vi "brookfield read external mode.vi"() -> ()   [LabVIEW 2019]
uses:
  <vilib>/Instr/_visa.llb/VISA Configure Serial Port (Instr).vi
panel:
  out "Conrtro Circuitry Enabled":bool
  out "Motor On":bool
  out "Motor Stopped":bool
  out "Auto-zero Complete":bool
  out "Motor Circuit Error":bool
  out "Diagnostics Error":bool
  out "Invalid Command Received":bool
  out "resulting string":string
  out "temp":dbl
  out "torque%":dbl
  out "length":i32
  out "read buffer":string
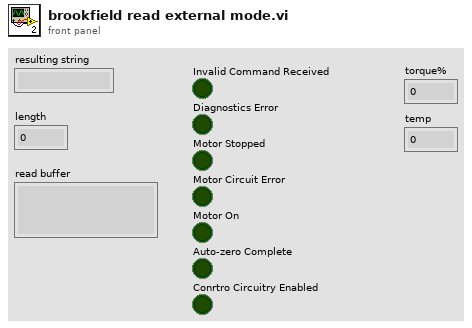
[diagram p1: front panel]
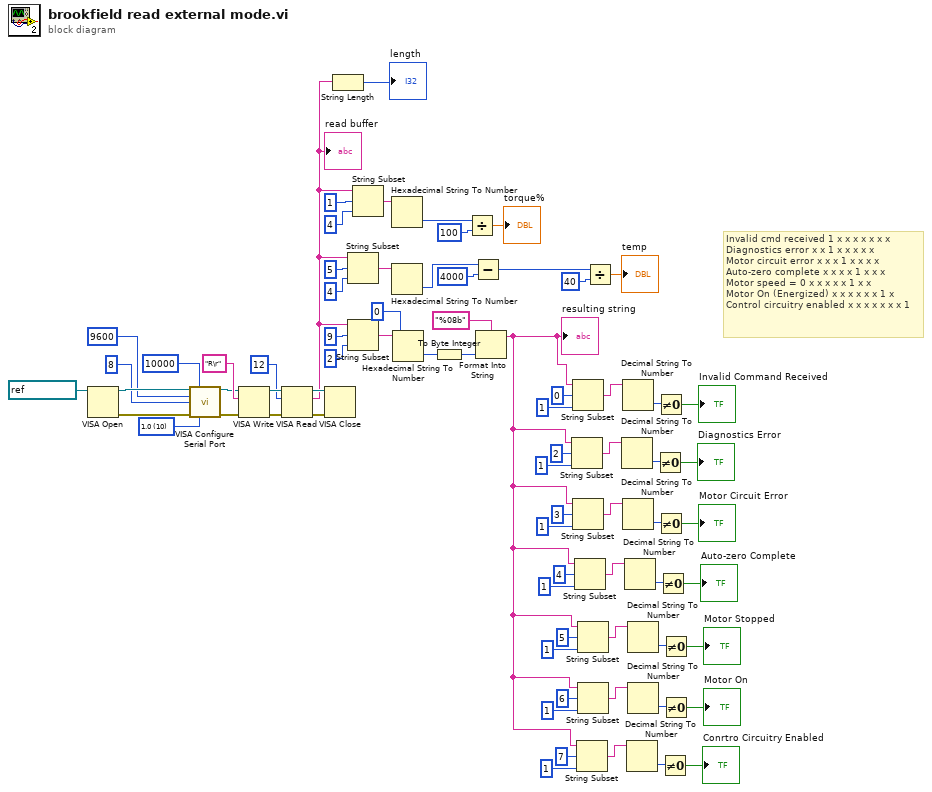
[diagram p0: block diagram]
diagram:
  w63 = u16 10 items=["1.0"=10, "1.5"=15, "2.0"=20] ("stop bits (10: 1 bit)")
  # "Invalid cmd received 1 x x x x x x x\nDiagnostics error x x 1 x x x x x\nMotor circuit error x x x 1 x x x x\nAuto-zero complete x x x x 1 x x x\nMotor speed = 0 x x x x x 1 x x\nMotor On (Energized) x x x x x x 1 x\nControl circuitry enabled x x x x x x x 1"
  n1 = VISA Open(VISA resource name=refnum<visa-resource-name> "COM11" ("Conductivity Port")) -> (VISA resource name=w67:refnum<visa-resource-name>, error out=w69:errorcluster)  [unwired: 4 in]
  n2 = call-poly "VISA Configure Serial Port"("VISA resource name"=w67, "timeout (10sec)"=u32 10000, "baud rate (9600)"=u32 9600, "data bits (8)"=u16 8, "error in (no error)"=w69, "stop bits (10: 1 bit)"=w63) -> ("VISA resource name out"=w62:refnum<visa-resource-name>, "error out"=w61:errorcluster)  [unwired: 8 in]
  n3 = VISA Write(VISA resource name=w62, write buffer="R\r", error in (no error)=w61) -> (VISA resource name out=w73:refnum<visa-resource-name>, error out=w72:errorcluster)  [unwired: 1 out]
  n4 = VISA Read(VISA resource name=w73, byte count=u32 12, error in (no error)=w72) -> (VISA resource name out=w60:refnum<visa-resource-name>, read buffer=w42:string, error out=w59:errorcluster)  [unwired: 1 out]
  "read buffer" <- w42
  n5 = VISA Close(VISA resource name=w60, error in (no error)=w59) -> ()  [unwired: 1 out]
  n6 = String Length(string=w42) -> (length=→"length":i32)
  n7 = String Subset(string=w42, offset (0)=5, length (rest)=4 ("length (rest)")) -> (substring=w49:string)
  n8 = String Subset(string=w42, offset (0)=9, length (rest)=2 ("length (rest)")) -> (substring=w41:string)
  n9 = String Subset(string=w42, offset (0)=1, length (rest)=4 ("length (rest)")) -> (substring=w56:string)
  n10 = Hexadecimal String To Number(string=w56) -> (number=w55:u32)  [unwired: 2 in, 1 out]
  n11 = Hexadecimal String To Number(string=w49) -> (number=w48:u32)  [unwired: 2 in, 1 out]
  n12 = Hexadecimal String To Number(string=w41, default (0uL)=u32 0 ("default (0 U32)")) -> (number=w32:u32)  [unwired: 1 in, 1 out]
  n13 = To Byte Integer(number=w32) -> (8bit integer=w33:i8)
  n14 = Divide(x=w55, y=u32 100) -> (x/y=→"torque%":dbl)
  n15 = Subtract(x=w48, y=u32 4000) -> (x-y=w46:u32)
  n16 = Format Into String(format string="%08b", w33) -> (resulting string=w1:string)  [unwired: 2 in, 1 out]
  "resulting string" <- w1
  n17 = String Subset(string=w1, offset (0)=2, length (rest)=1 ("length (rest)")) -> (substring=w29:string)
  n18 = String Subset(string=w1, offset (0)=0, length (rest)=1 ("length (rest)")) -> (substring=w37:string)
  n19 = String Subset(string=w1, offset (0)=3, length (rest)=1 ("length (rest)")) -> (substring=w24:string)
  n20 = String Subset(string=w1, offset (0)=4, length (rest)=1 ("length (rest)")) -> (substring=w19:string)
  n21 = String Subset(string=w1, offset (0)=7, length (rest)=1 ("length (rest)")) -> (substring=w4:string)
  n22 = String Subset(string=w1, offset (0)=5, length (rest)=1 ("length (rest)")) -> (substring=w14:string)
  n23 = String Subset(string=w1, offset (0)=6, length (rest)=1 ("length (rest)")) -> (substring=w9:string)
  n24 = Divide(x=w46, y=u32 40) -> (x/y=→"temp":dbl)
  n25 = Decimal String To Number(string=w29) -> (number=w30:i32)  [unwired: 2 in, 1 out]
  n26 = Decimal String To Number(string=w37) -> (number=w36:i32)  [unwired: 2 in, 1 out]
  n27 = Decimal String To Number(string=w24) -> (number=w23:i32)  [unwired: 2 in, 1 out]
  n28 = Decimal String To Number(string=w19) -> (number=w20:i32)  [unwired: 2 in, 1 out]
  n29 = Decimal String To Number(string=w4) -> (number=w3:i32)  [unwired: 2 in, 1 out]
  n30 = Decimal String To Number(string=w14) -> (number=w13:i32)  [unwired: 2 in, 1 out]
  n31 = Decimal String To Number(string=w9) -> (number=w10:i32)  [unwired: 2 in, 1 out]
  n32 = Not Equal To 0?(x=w30) -> (x != 0?=→"Diagnostics Error":bool)
  n33 = Not Equal To 0?(x=w36) -> (x != 0?=→"Invalid Command Received":bool)
  n34 = Not Equal To 0?(x=w23) -> (x != 0?=→"Motor Circuit Error":bool)
  n35 = Not Equal To 0?(x=w20) -> (x != 0?=→"Auto-zero Complete":bool)
  n36 = Not Equal To 0?(x=w3) -> (x != 0?=→"Conrtro Circuitry Enabled":bool)
  n37 = Not Equal To 0?(x=w13) -> (x != 0?=→"Motor Stopped":bool)
  n38 = Not Equal To 0?(x=w10) -> (x != 0?=→"Motor On":bool)
